vi "TCP_Module.vi"(8 "error in (no error)":errorcluster) -> (0 "error out":errorcluster)   [LabVIEW 2021]
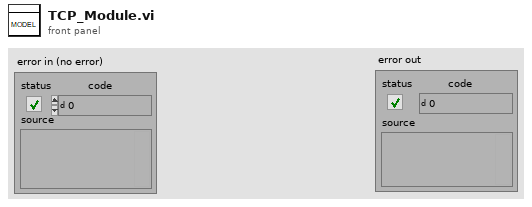
[diagram p1: front panel]
types:
  T1 = enum32{"Invalid", "Standard", "Closed", "Hidden", "Minimized", "Maximized"}
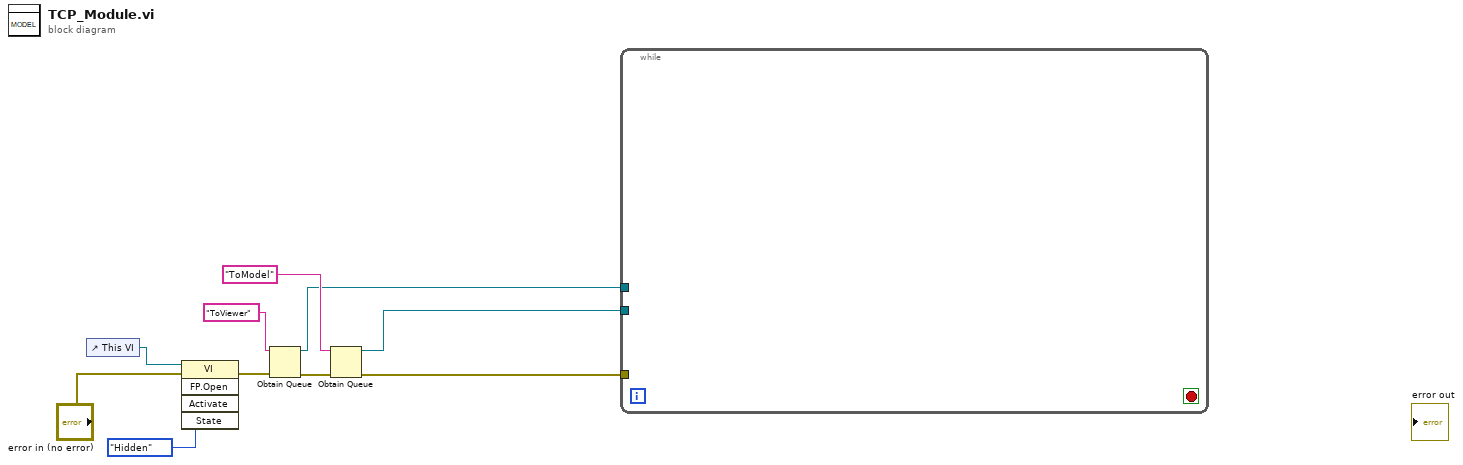
[diagram p0: block diagram]
diagram:
  n1 = control-ref of="This VI"() -> (w10:refnum<vi>)
  n2 = invoke class="VI" method="FP.Open"(reference=w10, error in="error in (no error)", "State"=T1."Hidden") -> (error out=w7:errorcluster)  [unwired: 2 in, 4 out]
  n3 = Obtain Queue(name (unnamed)="ToViewer", error in (no error)=w7) -> (queue out=w1:refnum<queue>, error out=w6:errorcluster)  [unwired: 3 in, 1 out]
  n4 = Obtain Queue(name (unnamed)="ToModel", error in (no error)=w6) -> (queue out=w2:refnum<queue>, error out=w4:errorcluster)  [unwired: 3 in, 1 out]
  n5 = while {
    tunnel: w4 -> [_]
    tunnel: w2 -> [_]
    tunnel: w1 -> [_]
    stop <- _ stop-if-true
  }
